vi "DisplayJson.vi"(11 "JSON String In":string="[{\"version\":\"1.0.0\",\"header\":{\"creationDate\":\"2022-06-03T00:00:00\",\"remarks\":\"\",\"serialNumber\":\"98172\",\"productNumber\":\"123021.1804\",\"productType\":\"PAA-9L\",\"pressureType\":2,\"productSeries\":\"9L\",\"compensatedTemperatureRange\":{\"min\":-10.0,\"max\":80.0,\"unit\":4},\"compensatedPressureRange\":{\"min\":0.0,\"max\":0.35,\"unit\":3},\"electricSupply\":{\"magnitude\":1.0,\"unit\":18},\"orderNumber\":9990266,\"orderPosition\":3,\"orderTargetDispatchDate\":\"2022-06-02T00:00:00+00:00\",\"customerName\":\"DemoData Inc.\",\"customerNumber\":12345678,\"customerOrderNumber\":\"Cust-9990266-123\",\"customerReferenceNumber\":\"\",\"customerProductT...") -> ()   [LabVIEW 2017] (continued)
{\"magnitude\":0.0013623391,\"unit\":7}},\"temperature\":{\"output\":{\"magnitude\":-10.8346,\"unit\":4},\"error\":{\"magnitude\":-0.10593532,\"unit\":4}}}}}},{\"reference\":\"F_12300_XX_0000098765\",\"environmentTarget\":{\"pressure\":{\"magnitude\":0.27,\"unit\":3},\"temperature\":{\"magnitude\":-10.0,\"unit\":4}},\"environment\":{\"pressure\":{\"magnitude\":0.270004,\"unit\":3},\"temperature\":{\"magnitude\":-10.7286,\"unit\":4},\"supply\":{\"magnitude\":1.0,\"unit\":18}},\"raw\":{\"signal\":{\"magnitude\":47.450500568,\"unit\":22},\"bridgeResistance\":{\"magnitude\":3280.1356798,\"unit\":28}},\"compensated\":{\"mathematicalModels\":{\"MM0123\":{\"pressure\":{\"output\":{\"magnitude\":0.27003,\"unit\":3},\"error\":{\"magnitude\":0.0074227521,\"unit\":7}},\"temperature\":{\"output\":{\"magnitude\":-10.8303,\"unit\":4},\"error\":{\"magnitude\":-0.10169503,\"unit\":4}}}}}},{\"reference\":\"F_12300_XX_0000098765\",\"environmentTarget\":{\"pressure\":{\"magnitude\":0.35,\"unit\":3},\"temperature\":{\"magnitude\":-10.0,\"unit\":4}},\"environment\":{\"pressure\":{\"magnitude\":0.350008,\"unit\":3},\"temperature\":{\"magnitude\":-10.7286,\"unit\":4},\"supply\":{\"magnitude\":1.0,\"unit\":18}},\"raw\":{\"signal\":{\"magnitude\":58.239105783,\"unit\":22},\"bridgeResistance\":{\"magnitude\":3276.3155459,\"unit\":28}},\"compensated\":{\"mathematicalModels\":{\"MM0123\":{\"pressure\":{\"output\":{\"magnitude\":0.350007,\"unit\":3},\"error\":{\"magnitude\":-0.00029844865,\"unit\":7}},\"temperature\":{\"output\":{\"magnitude\":-10.8321,\"unit\":4},\"error\":{\"magnitude\":-0.1035134,\"unit\":4}}}}}},{\"reference\":\"F_12300_XX_0000098765\",\"environmentTarget\":{\"pressure\":{\"magnitude\":0.03,\"unit\":3},\"temperature\":{\"magnitude\":0.0,\"unit\":4}},\"environment\":{\"pressure\":{\"magnitude\":0.0299972,\"unit\":3},\"temperature\":{\"magnitude\":-0.629962,\"unit\":4},\"supply\":{\"magnitude\":1.0,\"unit\":18}},\"raw\":{\"signal\":{\"magnitude\":15.244054572,\"unit\":22},\"bridgeResistance\":{\"magnitude\":3361.0174053,\"unit\":28}},\"compensated\":{\"mathematicalModels\":{\"MM0123\":{\"pressure\":{\"output\":{\"magnitude\":0.0300171,\"unit\":3},\"error\":{\"magnitude\":0.0056759296,\"unit\":7}},\"temperature\":{\"output\":{\"magnitude\":-0.733085,\"unit\":4},\"error\":{\"magnitude\":-0.10312274,\"unit\":4}}}}}},{\"reference\":\"F_12300_XX_0000098765\",\"environmentTarget\":{\"pressure\":{\"magnitude\":0.11,\"unit\":3},\"temperature\":{\"magnitude\":0.0,\"unit\":4}},\"environment\":{\"pressure\":{\"magnitude\":0.109991,\"unit\":3},\"temperature\":{\"magnitude\":-0.629962,\"unit\":4},\"supply\":{\"magnitude\":1.0,\"unit\":18}},\"raw\":{\"signal\":{\"magnitude\":26.124449139,\"unit\":22},\"bridgeResistance\":{\"magnitude\":3356.9112522,\"unit\":28}},\"compensated\":{\"mathematicalModels\":{\"MM0123\":{\"pressure\":{\"output\":{\"magnitude\":0.109967,\"unit\":3},\"error\":{\"magnitude\":-0.0069380952,\"unit\":7}},\"temperature\":{\"output\":{\"magnitude\":-0.737302,\"unit\":4},\"error\":{\"magnitude\":-0.10734013,\"unit\":4}}}}}},{\"reference\":\"F_12300_XX_0000098765\",\"environmentTarget\":{\"pressure\":{\"magnitude\":0.19,\"unit\":3},\"temperature\":{\"magnitude\":0.0,\"unit\":4}},\"environment\":{\"pressure\":{\"magnitude\":0.190002,\"unit\":3},\"temperature\":{\"magnitude\":-0.629962,\"unit\":4},\"supply\":{\"magnitude\":1.0,\"unit\":18}},\"raw\":{\"signal\":{\"magnitude\":36.977075789,\"unit\":22},\"bridgeResistance\":{\"magnitude\":3352.8969981,\"unit\":28}},\"compensated\":{\"mathematicalModels\":{\"MM0123\":{\"pressure\":{\"output\":{\"magnitude\":0.190006,\"unit\":3},\"error\":{\"magnitude\":0.0012306197,\"unit\":7}},\"temperature\":{\"output\":{\"magnitude\":-0.73875,\"unit\":4},\"error\":{\"magnitude\":-0.10878787,\"unit\":4}}}}}},{\"reference\":\"F_12300_XX_0000098765\",\"environmentTarget\":{\"pressure\":{\"magnitude\":0.27,\"unit\":3},\"temperature\":{\"magnitude\":0.0,\"unit\":4}},\"environment\":{\"pressure\":{\"magnitude\":0.269997,\"unit\":3},\"temperature\":{\"magnitude\":-0.629962,\"unit\":4},\"supply\":{\"magnitude\":1.0,\"unit\":18}},\"raw\":{\"signal\":{\"magnitude\":47.783782703,\"unit\":22},\"bridgeResistance\":{\"magnitude\":3348.9647898,\"unit\":28}},\"compensated\":{\"mathematicalModels\":{\"MM0123\":{\"pressure\":{\"output\":{\"magnitude\":0.270004,\"unit\":3},\"error\":{\"magnitude\":0.0019715764,\"unit\":7}},\"temperature\":{\"output\":{\"magnitude\":-0.74022,\"unit\":4},\"error\":{\"magnitude\":-0.11025793,\"unit\":4}}}}}},{\"reference\":\"F_12300_XX_0000098765\",\"environmentTarget\":{\"pressure\":{\"magnitude\":0.35,\"unit\":3},\"temperature\":{\"magnitude\":0.0,\"unit\":4}},\"environment\":{\"pressure\":{\"magnitude\":0.350002,\"unit\":3},\"temperature\":{\"magnitude\":-0.629962,\"unit\":4},\"supply\":{\"magnitude\":1.0,\"unit\":18}},\"raw\":{\"signal\":{\"magnitude\":58.546481606,\"unit\":22},\"bridgeResistance\":{\"magnitude\":3345.1070624,\"unit\":28}},\"compensated\":{\"mathematicalModels\":{\"MM0123\":{\"pressure\":{\"output\":{\"magnitude\":0.349974,\"unit\":3},\"error\":{\"magnitude\":-0.0079123893,\"unit\":7}},\"temperature\":{\"output\":{\"magnitude\":-0.743146,\"unit\":4},\"error\":{\"magnitude\":-0.11318368,\"unit\":4}}}}}},{\"reference\":\"F_12300_XX_0000098765\",\"environmentTarget\":{\"pressure\":{\"magnitude\":0.03,\"unit\":3},\"temperature\":{\"magnitude\":20.0,\"unit\":4}},\"environment\":{\"pressure\":{\"magnitude\":0.0300081,\"unit\":3},\"temperature\":{\"magnitude\":19.5509,\"unit\":4},\"supply\":{\"magnitude\":1.0,\"unit\":18}},\"raw\":{\"signal\":{\"magnitude\":16.125304957,\"unit\":22},\"bridgeResistance\":{\"magnitude\":3516.1742855,\"unit\":28}},\"compensated\":{\"mathematicalModels\":{\"MM0123\":{\"pressure\":{\"output\":{\"magnitude\":0.0300105,\"unit\":3},\"error\":{\"magnitude\":0.00067553345,\"unit\":7}},\"temperature\":{\"output\":{\"magnitude\":19.5453,\"unit\":4},\"error\":{\"magnitude\":-0.0056133347,\"unit\":4}}}}}},{\"reference\":\"F_12300_XX_0000098765\",\"environmentTarget\":{\"pressure\":{\"magnitude\":0.11,\"unit\":3},\"temperature\":{\"magnitude\":20.0,\"unit\":4}},\"environment\":{\"pressure\":{\"magnitude\":0.110005,\"unit\":3},\"temperature\":{\"magnitude\":19.5509,\"unit\":4},\"supply\":{\"magnitude\":1.0,\"unit\":18}},\"raw\":{\"signal\":{\"magnitude\":26.996372938,\"unit\":22},\"bridgeResistance\":{\"magnitude\":3512.074279,\"unit\":28}},\"compensated\":{\"mathematicalModels\":{\"MM0123\":{\"pressure\":{\"output\":{\"magnitude\":0.109981,\"unit\":3},\"error\":{\"magnitude\":-0.006982433,\"unit\":7}},\"temperature\":{\"output\":{\"magnitude\":19.5417,\"unit\":4},\"error\":{\"magnitude\":-0.0092010915,\"unit\":4}}}}}},{\"reference\":\"F_12300_XX_0000098765\",\"environmentTarget\":{\"pressure\":{\"magnitude\":0.19,\"unit\":3},\"temperature\":{\"magnitude\":20.0,\"unit\":4}},\"environment\":{\"pressure\":{\"magnitude\":0.19,\"unit\":3},\"temperature\":{\"magnitude\":19.5509,\"unit\":4},\"supply\":{\"magnitude\":1.0,\"unit\":18}},\"raw\":{\"signal\":{\"magnitude\":37.839811244,\"unit\":22},\"bridgeResistance\":{\"magnitude\":3508.0539307,\"unit\":28}},\"compensated\":{\"mathematicalModels\":{\"MM0123\":{\"pressure\":{\"output\":{\"magnitude\":0.190009,\"unit\":3},\"error\":{\"magnitude\":0.0025189522,\"unit\":7}},\"temperature\":{\"output\":{\"magnitude\":19.5397,\"unit\":4},\"error\":{\"magnitude\":-0.011265038,\"unit\":4}}}}}},{\"reference\":\"F_12300_XX_0000098765\",\"environmentTarget\":{\"pressure\":{\"magnitude\":0.27,\"unit\":3},\"temperature\":{\"magnitude\":20.0,\"unit\":4}},\"environment\":{\"pressure\":{\"magnitude\":0.269991,\"unit\":3},\"temperature\":{\"magnitude\":19.5509,\"unit\":4},\"supply\":{\"magnitude\":1.0,\"unit\":18}},\"raw\":{\"signal\":{\"magnitude\":48.64477597,\"unit\":22},\"bridgeResistance\":{\"magnitude\":3504.0815507,\"unit\":28}},\"compensated\":{\"mathematicalModels\":{\"MM0123\":{\"pressure\":{\"output\":{\"magnitude\":0.270017,\"unit\":3},\"error\":{\"magnitude\":0.0075196359,\"unit\":7}},\"temperature\":{\"output\":{\"magnitude\":19.5351,\"unit\":4},\"error\":{\"magnitude\":-0.015767596,\"unit\":4}}}}}},{\"reference\":\"F_12300_XX_0000098765\",\"environmentTarget\":{\"pressure\":{\"magnitude\":0.35,\"unit\":3},\"temperature\":{\"magnitude\":20.0,\"unit\":4}},\"environment\":{\"pressure\":{\"magnitude\":0.350006,\"unit\":3},\"temperature\":{\"magnitude\":19.5509,\"unit\":4},\"supply\":{\"magnitude\":1.0,\"unit\":18}},\"raw\":{\"signal\":{\"magnitude\":59.412702159,\"unit\":22},\"bridgeResistance\":{\"magnitude\":3500.1828661,\"unit\":28}},\"compensated\":{\"mathematicalModels\":{\"MM0123\":{\"pressure\":{\"output\":{\"magnitude\":0.350016,\"unit\":3},\"error\":{\"magnitude\":0.0028004951,\"unit\":7}},\"temperature\":{\"output\":{\"magnitude\":19.5311,\"unit\":4},\"error\":{\"magnitude\":-0.01974258,\"unit\":4}}}}}},{\"reference\":\"F_12300_XX_0000098765\",\"environmentTarget\":{\"pressure\":{\"magnitude\":0.03,\"unit\":3},\"temperature\":{\"magnitude\":40.0,\"unit\":4}},\"environment\":{\"pressure\":{\"magnitude\":0.0299895,\"unit\":3},\"temperature\":{\"magnitude\":39.7284,\"unit\":4},\"supply\":{\"magnitude\":1.0,\"unit\":18}},\"raw\":{\"signal\":{\"magnitude\":17.065348991,\"unit\":22},\"bridgeResistance\":{\"magnitude\":3692.0667607,\"unit\":28}},\"compensated\":{\"mathematicalModels\":{\"MM0123\":{\"pressure\":{\"output\":{\"magnitude\":0.0300063,\"unit\":3},\"error\":{\"magnitude\":0.0050974158,\"unit\":7}},\"temperature\":{\"output\":{\"magnitude\":39.7232,\"unit\":4},\"error\":{\"magnitude\":-0.0052473995,\"unit\":4}}}}}},{\"reference\":\"F_12300_XX_0000098765\",\"environmentTarget\":{\"pressure\":{\"magnitude\":0.11,\"unit\":3},\"temperature\":{\"magnitude\":40.0,\"unit\":4}},\"environment\":{\"pressure\":{\"magnitude\":0.110003,\"unit\":3},\"temperature\":{\"magnitude\":39.7284,\"unit\":4},\"supply\":{\"magnitude\":1.0,\"unit\":18}},\"raw\":{\"signal\":{\"magnitude\":27.983427862,\"unit\":22},\"bridgeResistance\":{\"magnitude\":3687.9377706,\"unit\":28}},\"compensated\":{\"mathematicalModels\":{\"MM0123\":{\"pressure\":{\"output\":{\"magnitude\":0.109977,\"unit\":3},\"error\":{\"magnitude\":-0.0073825952,\"unit\":7}},\"temperature\":{\"output\":{\"magnitude\":39.7238,\"unit\":4},\"error\":{\"magnitude\":-0.004664108,\"unit\":4}}}}}},{\"reference\":\"F_12300_XX_0000098765\",\"environmentTarget\":{\"pressure\":{\"magnitude\":0.19,\"unit\":3},\"temperature\":{\"magnitude\":40.0,\"unit\":4}},\"environment\":{\"pressure\":{\"magnitude\":0.190001,\"unit\":3},\"temperature\":{\"magnitude\":39.7284,\"unit\":4},\"supply\":{\"magnitude\":1.0,\"unit\":18}},\"raw\":{\"signal\":{\"magnitude\":38.877031412,\"unit\":22},\"bridgeResistance\":{\"magnitude\":3683.8203033,\"unit\":28}},\"compensated\":{\"mathematicalModels\":{\"MM0123\":{\"pressure\":{\"output\":{\"magnitude\":0.190002,\"unit\":3},\"error\":{\"magnitude\":0.00023079502,\"unit\":7}},\"temperature\":{\"output\":{\"magnitude\":39.7172,\"unit\":4},\"error\":{\"magnitude\":-0.011209563,\"unit\":4}}}}}},{\"reference\":\"F_12300_XX_0000098765\",\"environmentTarget\":{\"pressure\":{\"magnitude\":0.27,\"unit\":3},\"temperature\":{\"magnitude\":40.0,\"unit\":4}},\"environment\":{\"pressure\":{\"magnitude\":0.269992,\"unit\":3},\"temperature\":{\"magnitude\":39.7284,\"unit\":4},\"supply\":{\"magnitude\":1.0,\"unit\":18}},\"raw\":{\"signal\":{\"magnitude\":49.737147354,\"unit\":22},\"bridgeResistance\":{\"magnitude\":3679.8954018,\"unit\":28}},\"compensated\":{\"mathematicalModels\":{\"MM0123\":{\"pressure\":{\"output\":{\"magnitude\":0.270007,\"unit\":3},\"error\":{\"magnitude\":0.0041943925,\"unit\":7}},\"temperature\":{\"output\":{\"magnitude\":39.7218,\"unit\":4},\"error\":{\"magnitude\":-0.0066394556,\"unit\":4}}}}}},{\"reference\":\"F_12300_XX_0000098765\",\"environmentTarget\":{\"pressure\":{\"magnitude\":0.35,\"unit\":3},\"temperature\":{\"magnitude\":40.0,\"unit\":4}},\"environment\":{\"pressure\":{\"magnitude\":0.350005,\"unit\":3},\"temperature\":{\"magnitude\":39.7284,\"unit\":4},\"supply\":{\"magnitude\":1.0,\"unit\":18}},\"raw\":{\"signal\":{\"magnitude\":60.561192593,\"unit\":22},\"bridgeResistance\":{\"magnitude\":3675.9578376,\"unit\":28}},\"compensated\":{\"mathematicalModels\":{\"MM0123\":{\"pressure\":{\"output\":{\"magnitude\":0.34998,\"unit\":3},\"error\":{\"magnitude\":-0.0070559456,\"unit\":7}},\"temperature\":{\"output\":{\"magnitude\":39.7183,\"unit\":4},\"error\":{\"magnitude\":-0.010071361,\"unit\":4}}}}}},{\"reference\":\"F_12300_XX_0000098765\",\"environmentTarget\":{\"pressure\":{\"magnitude\":0.03,\"unit\":3},\"temperature\":{\"magnitude\":60.0,\"unit\":4}},\"environment\":{\"pressure\":{\"magnitude\":0.0299998,\"unit\":3},\"temperature\":{\"magnitude\":59.8651,\"unit\":4},\"supply\":{\"magnitude\":1.0,\"unit\":18}},\"raw\":{\"signal\":{\"magnitude\":18.099851195,\"unit\":22},\"bridgeResistance\":{\"magnitude\":3895.3174051,\"unit\":28}},\"compensated\":{\"mathematicalModels\":{\"MM0123\":{\"pressure\":{\"output\":{\"magnitude\":0.0300101,\"unit\":3},\"error\":{\"magnitude\":0.0029412823,\"unit\":7}},\"temperature\":{\"output\":{\"magnitude\":59.9224,\"unit\":4},\"error\":{\"magnitude\":0.057229128,\"unit\":4}}}}}},{\"reference\":\"F_12300_XX_0000098765\",\"environmentTarget\":{\"pressure\":{\"magnitude\":0.11,\"unit\":3},\"temperature\":{\"magnitude\":60.0,\"unit\":4}},\"environment\":{\"pressure\":{\"magnitude\":0.110001,\"unit\":3},\"temperature\":{\"magnitude\":59.8651,\"unit\":4},\"supply\":{\"magnitude\":1.0,\"unit\":18}},\"raw\":{\"signal\":{\"magnitude\":29.103136685,\"unit\":22},\"bridgeResistance\":{\"magnitude\":3891.1648478,\"unit\":28}},\"compensated\":{\"mathematicalModels\":{\"MM0123\":{\"pressure\":{\"output\":{\"magnitude\":0.109978,\"unit\":3},\"error\":{\"magnitude\":-0.0066748143,\"unit\":7}},\"temperature\":{\"output\":{\"magnitude\":59.9257,\"unit\":4},\"error\":{\"magnitude\":0.06060745,\"unit\":4}}}}}},{\"reference\":\"F_12300_XX_0000098765\",\"environmentTarget\":{\"pressure\":{\"magnitude\":0.19,\"unit\":3},\"temperature\":{\"magnitude\":60.0,\"unit\":4}},\"environment\":{\"pressure\":{\"magnitude\":0.190003,\"unit\":3},\"temperature\":{\"magnitude\":59.8651,\"unit\":4},\"supply\":{\"magnitude\":1.0,\"unit\":18}},\"raw\":{\"signal\":{\"magnitude\":40.086606504,\"unit\":22},\"bridgeResistance\":{\"magnitude\":3877.0460541,\"unit\":28}},\"compensated\":{\"mathematicalModels\":{\"MM0123\":{\"pressure\":{\"output\":{\"magnitude\":0.190005,\"unit\":3},\"error\":{\"magnitude\":0.00046457429,\"unit\":7}},\"temperature\":{\"output\":{\"magnitude\":59.9272,\"unit\":4},\"error\":{\"magnitude\":0.062116452,\"unit\":4}}}}}},{\"reference\":\"F_12300_XX_0000098765\",\"environmentTarget\":{\"pressure\":{\"magnitude\":0.27,\"unit\":3},\"temperature\":{\"magnitude\":60.0,\"unit\":4}},\"environment\":{\"pressure\":{\"magnitude\":0.270002,\"unit\":3},\"temperature\":{\"magnitude\":59.8651,\"unit\":4},\"supply\":{\"magnitude\":1.0,\"unit\":18}},\"raw\":{\"signal\":{\"magnitude\":51.041325527,\"unit\":22},\"bridgeResistance\":{\"magnitude\":3872.9540114,\"unit\":28}},\"compensated\":{\"mathematicalModels\":{\"MM0123\":{\"pressure\":{\"output\":{\"magnitude\":0.270027,\"unit\":3},\"error\":{\"magnitude\":0.0071406806,\"unit\":7}},\"temperature\":{\"output\":{\"magnitude\":59.9256,\"unit\":4},\"error\":{\"magnitude\":0.060455959,\"unit\":4}}}}}},{\"reference\":\"F_12300_XX_0000098765\",\"environmentTarget\":{\"pressure\":{\"magnitude\":0.35,\"unit\":3},\"temperature\":{\"magnitude\":60.0,\"unit\":4}},\"environment\":{\"pressure\":{\"magnitude\":0.349997,\"unit\":3},\"temperature\":{\"magnitude\":59.8651,\"unit\":4},\"supply\":{\"magnitude\":1.0,\"unit\":18}},\"raw\":{\"signal\":{\"magnitude\":61.960627471,\"unit\":22},\"bridgeResistance\":{\"magnitude\":3868.9899215,\"unit\":28}},\"compensated\":{\"mathematicalModels\":{\"MM0123\":{\"pressure\":{\"output\":{\"magnitude\":0.349991,\"unit\":3},\"error\":{\"magnitude\":-0.0017872561,\"unit\":7}},\"temperature\":{\"output\":{\"magnitude\":59.9305,\"unit\":4},\"error\":{\"magnitude\":0.065332416,\"unit\":4}}}}}},{\"reference\":\"F_12300_XX_0000098765\",\"environmentTarget\":{\"pressure\":{\"magnitude\":0.03,\"unit\":3},\"temperature\":{\"magnitude\":80.0,\"unit\":4}},\"environment\":{\"pressure\":{\"magnitude\":0.0300094,\"unit\":3},\"temperature\":{\"magnitude\":79.9513,\"unit\":4},\"supply\":{\"magnitude\":1.0,\"unit\":18}},\"raw\":{\"signal\":{\"magnitude\":19.261952971,\"unit\":22},\"bridgeResistance\":{\"magnitude\":4092.4016691,\"unit\":28}},\"compensated\":{\"mathematicalModels\":{\"MM0123\":{\"pressure\":{\"output\":{\"magnitude\":0.0300217,\"unit\":3},\"error\":{\"magnitude\":0.0035217854,\"unit\":7}},\"temperature\":{\"output\":{\"magnitude\":80.0395,\"unit\":4},\"error\":{\"magnitude\":0.089127618,\"unit\":4}}}}}},{\"reference\":\"F_12300_XX_0000098765\",\"environmentTarget\":{\"pressure\":{\"magnitude\":0.11,\"unit\":3},\"temperature\":{\"magnitude\":80.0,\"unit\":4}},\"environment\":{\"pressure\":{\"magnitude\":0.109996,\"unit\":3},\"temperature\":{\"magnitude\":79.9513,\"unit\":4},\"supply\":{\"magnitude\":1.0,\"unit\":18}},\"raw\":{\"signal\":{\"magnitude\":30.373856674,\"unit\":22},\"bridgeResistance\":{\"magnitude\":4089.1956244,\"unit\":28}},\"compensated\":{\"mathematicalModels\":{\"MM0123\":{\"pressure\":{\"output\":{\"magnitude\":0.109968,\"unit\":3},\"error\":{\"magnitude\":-0.0080606507,\"unit\":7}},\"temperature\":{\"output\":{\"magnitude\":80.0443,\"unit\":4},\"error\":{\"magnitude\":0.093001611,\"unit\":4}}}}}},{\"reference\":\"F_12300_XX_0000098765\",\"environmentTarget\":{\"pressure\":{\"magnitude\":0.19,\"unit\":3},\"temperature\":{\"magnitude\":80.0,\"unit\":4}},\"environment\":{\"pressure\":{\"magnitude\":0.189998,\"unit\":3},\"temperature\":{\"magnitude\":79.9513,\"unit\":4},\"supply\":{\"magnitude\":1.0,\"unit\":18}},\"raw\":{\"signal\":{\"magnitude\":41.474863124,\"unit\":22},\"bridgeResistance\":{\"magnitude\":4084.0346992,\"unit\":28}},\"compensated\":{\"mathematicalModels\":{\"MM0123\":{\"pressure\":{\"output\":{\"magnitude\":0.190001,\"unit\":3},\"error\":{\"magnitude\":0.00091335112,\"unit\":7}},\"temperature\":{\"output\":{\"magnitude\":80.0507,\"unit\":4},\"error\":{\"magnitude\":0.099395557,\"unit\":4}}}}}},{\"reference\":\"F_12300_XX_0000098765\",\"environmentTarget\":{\"pressure\":{\"magnitude\":0.27,\"unit\":3},\"temperature\":{\"magnitude\":80.0,\"unit\":4}},\"environment\":{\"pressure\":{\"magnitude\":0.270001,\"unit\":3},\"temperature\":{\"magnitude\":79.9513,\"unit\":4},\"supply\":{\"magnitude\":1.0,\"unit\":18}},\"raw\":{\"signal\":{\"magnitude\":52.55093942,\"unit\":22},\"bridgeResistance\":{\"magnitude\":4079.8926343,\"unit\":28}},\"compensated\":{\"mathematicalModels\":{\"MM0123\":{\"pressure\":{\"output\":{\"magnitude\":0.270025,\"unit\":3},\"error\":{\"magnitude\":0.0067335623,\"unit\":7}},\"temperature\":{\"output\":{\"magnitude\":80.0559,\"unit\":4},\"error\":{\"magnitude\":0.10459769,\"unit\":4}}}}}},{\"reference\":\"F_12300_XX_0000098765\",\"environmentTarget\":{\"pressure\":{\"magnitude\":0.35,\"unit\":3},\"temperature\":{\"magnitude\":80.0,\"unit\":4}},\"environment\":{\"pressure\":{\"magnitude\":0.349998,\"unit\":3},\"temperature\":{\"magnitude\":79.9513,\"unit\":4},\"supply\":{\"magnitude\":1.0,\"unit\":18}},\"raw\":{\"signal\":{\"magnitude\":63.594920576,\"unit\":22},\"bridgeResistance\":{\"magnitude\":4075.8019906,\"unit\":28}},\"compensated\":{\"mathematicalModels\":{\"MM0123\":{\"pressure\":{\"output\":{\"magnitude\":0.349986,\"unit\":3},\"error\":{\"magnitude\":-0.0033814904,\"unit\":7}},\"temperature\":{\"output\":{\"magnitude\":80.0629,\"unit\":4},\"error\":{\"magnitude\":0.11256229,\"unit\":4}}}}}}]},{\"version\":\"1.0.0\",\"header\":{\"creationDate\":\"2022-06-03T00:00:00\",\"remarks\":\"\",\"serialNumber\":\"98153\",\"productNumber\":\"123021.1804\",\"productType\":\"PAA-9L\",\"pressureType\":2,\"productSeries\":\"9L\",\"compensatedTemperatureRange\":{\"min\":-10.0,\"max\":80.0,\"unit\":4},\"compensatedPressureRange\":{\"min\":0.0,\"max\":0.35,\"unit\":3},\"electricSupply\":{\"magnitude\":1.0,\"unit\":18},\"orderNumber\":9990266,\"orderPosition\":3,\"orderTargetDispatchDate\":\"2022-06-02T00:00:00+00:00\",\"customerName\":\"DemoData Inc.\",\"customerNumber\":12345678,\"customerOrderNumber\":\"Cust-9990266-123\",\"customerReferenceNumber\":\"\",\"customerProductType\":\"123021-1804 Rev.AA\"},\"compensationMethods\":{\"mathematicalModels\":{\"MM0123\":{\"modelType\":\"MM0123\",\"productNumber\":\"000000.0000\",\"compensatedTemperatureRange\":{\"min\":-10.0,\"max\":80.0,\"unit\":4},\"compensatedPressureRange\":{\"min\":0.0,\"max\":0.35,\"unit\":3},\"electricSupply\":{\"magnitude\":1.0,\"unit\":18},\"parts\":{\"pressure\":{\"inputs\":[\"Sig\",\"R\"],\"output\":\"P\",\"description\":\"P = f(Sig,R)\",\"coefficients\":[[5.01122025899,-0.00519005490227,1.99550532962E-06,-3.43406774518E-10,2.21550439359E-14],[-0.171430315338,0.000185608282359,-7.21762353561E-08,1.24734741497E-11,-8.09638944557E-16],[0.000333004920618,-3.38999107989E-07,1.30333721973E-10,-2.23231987141E-14,1.43329122857E-18]]},\"temperature\":{\"inputs\":[\"R\",\"Sig\"],\"output\":\"T\",\"description\":\"T = f(R,Sig)\",\"coefficients\":[[-8284.8728292,22.2690862439,-0.234676407299],[8.1751505771,-0.0232330277136,0.000254914377044],[-0.00308977224278,9.12200639172E-06,-1.03722430757E-07],[5.28453653046E-07,-1.59349229999E-09,1.87313443194E-11],[-3.40890563183E-11,1.04421357223E-13,-1.26657877517E-15]]}}}}},\"measurements\":[{\"reference\":\"F_12300_XX_0000098765\",\"environmentTarget\":{\"pressure\":{\"magnitude\":0.03,\"unit\":3},\"temperature\":{\"magnitude\":-10.0,\"unit\":4}},\"environment\":{\"pressure\":{\"magnitude\":0.0299989,\"unit\":3},\"temperature\":{\"magnitude\":-10.7286,\"unit\":4},\"supply\":{\"magnitude\":1.0,\"unit\":18}},\"raw\":{\"signal\":{\"magnitude\":17.244978392,\"unit\":22},\"bridgeResistance\":{\"magnitude\":3262.0216448,\"unit\":28}},\"compensated\":{\"mathematicalModels\":{\"MM0123\":{\"pressure\":{\"output\":{\"magnitude\":0.0300081,\"unit\":3},\"error\":{\"magnitude\":0.0026236255,\"unit\":7}},\"temperature\":{\"output\":{\"magnitude\":-10.8422,\"unit\":4},\"error\":{\"magnitude\":-0.11354536,\"unit\":4}}}}}},{\"reference\":\"F_12300_XX_0000098765\",\"environmentTarget\":{\"pressure\":{\"magnitude\":0.11,\"unit\":3},\"temperature\":{\"magnitude\":-10.0,\"unit\":4}},\"environment\":{\"pressure\":{\"magnitude\":0.109995,\"unit\":3},\"temperature\":{\"magnitude\":-10.7286,\"unit\":4},\"supply\":{\"magnitude\":1.0,\"unit\":18}},\"raw\":{\"signal\":{\"magnitude\":28.068610601,\"unit\":22},\"bridgeResistance\":{\"magnitude\":3257.9781268,\"unit\":28}},\"compensated\":{\"mathematicalModels\":{\"MM0123\":{\"pressure\":{\"output\":{\"magnitude\":0.109969,\"unit\":3},\"error\":{\"magnitude\":-0.0075611348,\"unit\":7}},\"temperature\":{\"output\":{\"magnitude\":-10.8372,\"unit\":4},\"error\":{\"magnitude\":-0.10860353,\"unit\":4}}}}}},{\"reference\":\"F_12300_XX_0000098765\",\"environmentTarget\":{\"pressure\":{\"magnitude\":0.19,\"unit\":3},\"temperature\":{\"magnitude\":-10.0,\"unit\":4}},\"environment\":{\"pressure\":{\"magnitude\":0.190006,\"unit\":3},\"temperature\":{\"magnitude\":-10.7286,\"unit\":4},\"supply\":{\"magnitude\":1.0,\"unit\":18}},\"raw\":{\"signal\":{\"magnitude\":38.861396244,\"unit\":22},\"bridgeResistance\":{\"magnitude\":3253.9392,\"unit\":28}},\"compensated\":{\"mathematicalModels\":{\"MM0123\":{\"pressure\":{\"output\":{\"magnitude\":0.190014,\"unit\":3},\"error\":{\"magnitude\":0.0022942891,\"unit\":7}},\"temperature\":{\"output\":{\"magnitude\":-10.8453,\"unit\":4},\"error\":{\"magnitude\":-0.11664439,\"unit\":4}}}}}},{\"reference\":\"F_12300_XX_0000098765\",\"environmentTarget\":{\"pressure\":{\"magnitude\":0.27,\"unit\":3},\"temperature\":{\"magnitude\":-10.0,\"unit\":4}},\"environment\":{\"pressure\":{\"magnitude\":0.270007,\"unit\":3},\"temperature\":{\"magnitude\":-10.7286,\"unit\":4},\"supply\":{\"magnitude\":1.0,\"unit\":18}},\"raw\":{\"signal\":{\"magnitude\":49.608942701,\"unit\":22},\"bridgeResistance\":{\"magnitude\":3250.0878585,\"unit\":28}},\"compensated\":{\"mathematicalModels\":{\"MM0123\":{\"pressure\":{\"output\":{\"magnitude\":0.270032,\"unit\":3},\"error\":{\"magnitude\":0.0071075807,\"unit\":7}},\"temperature\":{\"output\":{\"magnitude\":-10.84,\"unit\":4},\"error\":{\"magnitude\":-0.11234415,\"unit\":4}}}}}},{\"reference\":\"F_12300_XX_0000098765\",\"environmentTarget\":{\"pressure\":{\"magnitude\":0.35,\"unit\":3},\"temperature\":{\"magnitude\":-10.0,\"unit\":4}},\"environment\":{\"pressure\":{\"magnitude\":0.350003,\"unit\":3},\"temperature\":{\"magnitude\":-10.7286,\"unit\":4},\"supply\":{\"magnitude\":1.0,\"unit\":18}},\"raw\":{\"signal\":{\"magnitude\":60.306965463,\"unit\":22},\"bridgeResistance\":{\"magnitude\":3246.287526,\"unit\":28}},\"compensated\":{\"mathematicalModels\":{\"MM0123\":{\"pressure\":{\"output\":{\"magnitude\":0.35,\"unit\":3},\"error\":{\"magnitude\":-0.00094624232,\"unit\":7}},\"temperature\":{\"output\":{\"magnitude\":-10.8431,\"unit\":4},\"error\":{\"magnitude\":-0.11441768,\"unit\":4}}}}}},{\"reference\":\"F_12300_XX_0000098765\",\"environmentTarget\":{\"pressure\":{\"magnitude\":0.03,\"unit\":3},\"temperature\":{\"magnitude\":0.0,\"unit\":4}},\"environment\":{\"pressure\":{\"magnitude\":0.0299957,\"unit\":3},\"temperature\":{\"magnitude\":-0.629962,\"unit\":4},\"supply\":{\"magnitude\":1.0,\"unit\":18}},\"raw\":{\"signal\":{\"magnitude\":17.697410923,\"unit\":22},\"bridgeResistance\":{\"magnitude\":3330.8433823,\"unit\":28}},\"compensated\":{\"mathematicalModels\":{\"MM0123\":{\"pressure\":{\"output\":{\"magnitude\":0.0300103,\"unit\":3},\"error\":{\"magnitude\":0.0041629875,\"unit\":7}},\"temperature\":{\"output\":{\"magnitude\":-0.740686,\"unit\":4},\"error\":{\"magnitude\":-0.11072407,\"unit\":4}}}}}},{\"reference\":\"F_12300_XX_0000098765\",\"environmentTarget\":{\"pressure\":{\"magnitude\":0.11,\"unit\":3},\"temperature\":{\"magnitude\":0.0,\"unit\":4}},\"environment\":{\"pressure\":{\"magnitude\":0.109989,\"unit\":3},\"temperature\":{\"magnitude\":-0.629962,\"unit\":4},\"supply\":{\"magnitude\":1.0,\"unit\":18}},\"raw\":{\"signal\":{\"magnitude\":28.4892745,\"unit\":22},\"bridgeResistance\":{\"magnitude\":3326.7612608,\"unit\":28}},\"compensated\":{\"mathematicalModels\":{\"MM0123\":{\"pressure\":{\"output\":{\"magnitude\":0.109964,\"unit\":3},\"error\":{\"magnitude\":-0.0070954752,\"unit\":7}},\"temperature\":{\"output\":{\"magnitude\":-0.747272,\"unit\":4},\"error\":{\"magnitude\":-0.11731048,\"unit\":4}}}}}},{\"reference\":\"F_12300_XX_0000098765\",\"environmentTarget\":{\"pressure\":{\"magnitude\":0.19,\"unit\":3},\"temperature\":{\"magnitude\":0.0,\"unit\":4}},\"environment\":{\"pressure\":{\"magnitude\":0.190002,\"unit\":3},\"temperature\":{\"magnitude\":-0.629962,\"unit\":4},\"supply\":{\"magnitude\":1.0,\"unit\":18}},\"raw\":{\"signal\":{\"magnitude\":39.252857819,\"unit\":22},\"bridgeResistance\":{\"magnitude\":3322.8054195,\"unit\":28}},\"compensated\":{\"mathematicalModels\":{\"MM0123\":{\"pressure\":{\"output\":{\"magnitude\":0.189998,\"unit\":3},\"error\":{\"magnitude\":-0.0011297609,\"unit\":7}},\"temperature\":{\"output\":{\"magnitude\":-0.746289,\"unit\":4},\"error\":{\"magnitude\":-0.11632608,\"unit\":4}}}}}},{\"reference\":\"F_12300_XX_0000098765\",\"environmentTarget\":{\"pressure\":{\"magnitude\":0.27,\"unit\":3},\"temperature\":{\"magnitude\":0.0,\"unit\":4}},\"environment\":{\"pressure\":{\"magnitude\":0.269998,\"unit\":3},\"temperature\":{\"magnitude\":-0.629962,\"unit\":4},\"supply\":{\"magnitude\":1.0,\"unit\":18}},\"raw\":{\"signal\":{\"magnitude\":49.973804513,\"unit\":22},\"bridgeResistance\":{\"magnitude\":3318.899856,\"unit\":28}},\"compensated\":{\"mathematicalModels\":{\"MM0123\":{\"pressure\":{\"output\":{\"magnitude\":0.27001,\"unit\":3},\"error\":{\"magnitude\":0.0034989265,\"unit\":7}},\"temperature\":{\"output\":{\"magnitude\":-0.749528,\"unit\":4},\"error\":{\"magnitude\":-0.11956623,\"unit\":4}}}}}},{\"reference\":\"F_12300_XX_0000098765\",\"environmentTarget\":{\"pressure\":{\"magnitude\":0.35,\"unit\":3},\"temperature\":{\"magnitude\":0.0,\"unit\":4}},\"environment\":{\"pressure\":{\"magnitude\":0.350006,\"unit\":3},\"temperature\":{\"magnitude\":-0.629962,\"unit\":4},\"supply\":{\"magnitude\":1.0,\"unit\":18}},\"raw\":{\"signal\":{\"magnitude\":60.649198409,\"unit\":22},\"bridgeResistance\":{\"magnitude\":3315.0808233,\"unit\":28}},\"compensated\":{\"mathematicalModels\":{\"MM0123\":{\"pressure\":{\"output\":{\"magnitude\":0.349978,\"unit\":3},\"error\":{\"magnitude\":-0.0079789618,\"unit\":7}},\"temperature\":{\"output\":{\"magnitude\":-0.752383,\"unit\":4},\"error\":{\"magnitude\":-0.12242084,\"unit\":4}}}}}},{\"reference\":\"F_12300_XX_0000098765\",\"environmentTarget\":{\"pressure\":{\"magnitude\":0.03,\"unit\":3},\"temperature\":{\"magnitude\":20.0,\"unit\":4}},\"environment\":{\"pressure\":{\"magnitude\":0.029999,\"unit\":3},\"temperature\":{\"magnitude\":19.5509,\"unit\":4},\"supply\":{\"magnitude\":1.0,\"unit\":18}},\"raw\":{\"signal\":{\"magnitude\":18.650570403,\"unit\":22},\"bridgeResistance\":{\"magnitude\":3485.7702276,\"unit\":28}},\"compensated\":{\"mathematicalModels\":{\"MM0123\":{\"pressure\":{\"output\":{\"magnitude\":0.0300063,\"unit\":3},\"error\":{\"magnitude\":0.0020803458,\"unit\":7}},\"temperature\":{\"output\":{\"magnitude\":19.5415,\"unit\":4},\"error\":{\"magnitude\":-0.0093833592,\"unit\":4}}}}}},{\"reference\":\"F_12300_XX_0000098765\",\"environmentTarget\":{\"pressure\":{\"magnitude\":0.11,\"unit\":3},\"temperature\":{\"magnitude\":20.0,\"unit\":4}},\"environment\":{\"pressure\":{\"magnitude\":0.110002,\"unit\":3},\"temperature\":{\"magnitude\":19.5509,\"unit\":4},\"supply\":{\"magnitude\":1.0,\"unit\":18}},\"raw\":{\"signal\":{\"magnitude\":29.437602066,\"unit\":22},\"bridgeResistance\":{\"magnitude\":3481.7140234,\"unit\":28}},\"compensated\":{\"mathematicalModels\":{\"MM0123\":{\"pressure\":{\"output\":{\"magnitude\":0.109982,\"unit\":3},\"error\":{\"magnitude\":-0.0057937112,\"unit\":7}},\"temperature\":{\"output\":{\"magnitude\":19.5392,\"unit\":4},\"error\":{\"magnitude\":-0.011651533,\"unit\":4}}}}}},{\"reference\":\"F_12300_XX_0000098765\",\"environmentTarget\":{\"pressure\":{\"magnitude\":0.19,\"unit\":3},\"temperature\":{\"magnitude\":20.0,\"unit\":4}},\"environment\":{\"pressure\":{\"magnitude\":0.190002,\"unit\":3},\"temperature\":{\"magnitude\":19.5509,\"unit\":4},\"supply\":{\"magnitude\":1.0,\"unit\":18}},\"raw\":{\"signal\":{\"magnitude\":40.196372991,\"unit\":22},\"bridgeResistance\":{\"magnitude\":3477.715328,\"unit\":28}},\"compensated\":{\"mathematicalModels\":{\"MM0123\":{\"pressure\":{\"output\":{\"magnitude\":0.19001,\"unit\":3},\"error\":{\"magnitude\":0.0023661198,\"unit\":7}},\"temperature\":{\"output\":{\"magnitude\":19.5357,\"unit\":4},\"error\":{\"magnitude\":-0.015193505,\"unit\":4}}}}}},{\"reference\":\"F_12300_XX_0000098765\",\"environmentTarget\":{\"pressure\":{\"magnitude\":0.27,\"unit\":3},\"temperature\":{\"magnitude\":20.0,\"unit\":4}},\"environment\":{\"pressure\":{\"magnitude\":0.269995,\"unit\":3},\"temperature\":{\"magnitude\":19.5509,\"unit\":4},\"supply\":{\"magnitude\":1.0,\"unit\":18}},\"raw\":{\"signal\":{\"magnitude\":50.917814334,\"unit\":22},\"bridgeResistance\":{\"magnitude\":3473.7940622,\"unit\":28}},\"compensated\":{\"mathematicalModels\":{\"MM0123\":{\"pressure\":{\"output\":{\"magnitude\":0.270024,\"unit\":3},\"error\":{\"magnitude\":0.0082649059,\"unit\":7}},\"temperature\":{\"output\":{\"magnitude\":19.5329,\"unit\":4},\"error\":{\"magnitude\":-0.017941357,\"unit\":4}}}}}},{\"reference\":\"F_12300_XX_0000098765\",\"environmentTarget\":{\"pressure\":{\"magnitude\":0.35,\"unit\":3},\"temperature\":{\"magnitude\":20.0,\"unit\":4}},\"environment\":{\"pressure\":{\"magnitude\":0.350007,\"unit\":3},\"temperature\":{\"magnitude\":19.5509,\"unit\":4},\"supply\":{\"magnitude\":1.0,\"unit\":18}},\"raw\":{\"signal\":{\"magnitude\":61.600753754,\"unit\":22},\"bridgeResistance\":{\"magnitude\":3469.9282528,\"unit\":28}},\"compensated\":{\"mathematicalModels\":{\"MM0123\":{\"pressure\":{\"output\":{\"magnitude\":0.350015,\"unit\":3},\"error\":{\"magnitude\":0.002212532,\"unit\":7}},\"temperature\":{\"output\":{\"magnitude\":19.5283,\"unit\":4},\"error\":{\"magnitude\":-0.022578737,\"unit\":4}}}}}},{\"reference\":\"F_12300_XX_0000098765\",\"environmentTarget\":{\"pressure\":{\"magnitude\":0.03,\"unit\":3},\"temperature\":{\"magnitude\":40.0,\"unit\":4}},\"environment\":{\"pressure\":{\"magnitude\":0.0300029,\"unit\":3},\"temperature\":{\"magnitude\":39.7284,\"unit\":4},\"supply\":{\"magnitude\":1.0,\"unit\":18}},\"raw\":{\"signal\":{\"magnitude\":19.689183227,\"unit\":22},\"bridgeResistance\":{\"magnitude\":3660.9751606,\"unit\":28}},\"compensated\":{\"mathematicalModels\":{\"MM0123\":{\"pressure\":{\"output\":{\"magnitude\":0.0300171,\"unit\":3},\"error\":{\"magnitude\":0.004062793,\"unit\":7}},\"temperature\":{\"output\":{\"magnitude\":39.7238,\"unit\":4},\"error\":{\"magnitude\":-0.0046353676,\"unit\":4}}}}}},{\"reference\":\"F_12300_XX_0000098765\",\"environmentTarget\":{\"pressure\":{\"magnitude\":0.11,\"unit\":3},\"temperature\":{\"magnitude\":40.0,\"unit\":4}},\"environment\":{\"pressure\":{\"magnitude\":0.110002,\"unit\":3},\"temperature\":{\"magnitude\":39.7284,\"unit\":4},\"supply\":{\"magnitude\":1.0,\"unit\":18}},\"raw\":{\"signal\":{\"magnitude\":30.524706124,\"unit\":22},\"bridgeResistance\":{\"magnitude\":3656.8762185,\"unit\":28}},\"compensated\":{\"mathematicalModels\":{\"MM0123\":{\"pressure\":{\"output\":{\"magnitude\":0.109977,\"unit\":3},\"error\":{\"magnitude\":-0.0071312014,\"unit\":7}},\"temperature\":{\"output\":{\"magnitude\":39.7238,\"unit\":4},\"error\":{\"magnitude\":-0.0045700104,\"unit\":4}}}}}},{\"reference\":\"F_12300_XX_0000098765\",\"environmentTarget\":{\"pressure\":{\"magnitude\":0.19,\"unit\":3},\"temperature\":{\"magnitude\":40.0,\"unit\":4}},\"environment\":{\"pressure\":{\"magnitude\":0.190005,\"unit\":3},\"temperature\":{\"magnitude\":39.7284,\"unit\":4},\"supply\":{\"magnitude\":1.0,\"unit\":18}},\"raw\":{\"signal\":{\"magnitude\":41.337078939,\"unit\":22},\"bridgeResistance\":{\"magnitude\":3652.7974978,\"unit\":28}},\"compensated\":{\"mathematicalModels\":{\"MM0123\":{\"pressure\":{\"output\":{\"magnitude\":0.190002,\"unit\":3},\"error\":{\"magnitude\":-0.00072364867,\"unit\":7}},\"temperature\":{\"output\":{\"magnitude\":39.718,\"unit\":4},\"error\":{\"magnitude\":-0.0103739,\"unit\":4}}}}}},{\"reference\":\"F_12300_XX_0000098765\",\"environmentTarget\":{\"pressure\":{\"magnitude\":0.27,\"unit\":3},\"temperature\":{\"magnitude\":40.0,\"unit\":4}},\"environment\":{\"pressure\":{\"magnitude\":0.269992,\"unit\":3},\"temperature\":{\"magnitude\":39.7284,\"unit\":4},\"supply\":{\"magnitude\":1.0,\"unit\":18}},\"raw\":{\"signal\":{\"magnitude\":52.115466737,\"unit\":22},\"bridgeResistance\":{\"magnitude\":3648.891645,\"unit\":28}},\"compensated\":{\"mathematicalModels\":{\"MM0123\":{\"pressure\":{\"output\":{\"magnitude\":0.270006,\"unit\":3},\"error\":{\"magnitude\":0.004101221,\"unit\":7}},\"temperature\":{\"output\":{\"magnitude\":39.7215,\"unit\":4},\"error\":{\"magnitude\":-0.0068958529,\"unit\":4}}}}}},{\"reference\":\"F_12300_XX_0000098765\",\"environmentTarget\":{\"pressure\":{\"magnitude\":0.35,\"unit\":3},\"temperature\":{\"magnitude\":40.0,\"unit\":4}},\"environment\":{\"pressure\":{\"magnitude\":0.350002,\"unit\":3},\"temperature\":{\"magnitude\":39.7284,\"unit\":4},\"supply\":{\"magnitude\":1.0,\"unit\":18}},\"raw\":{\"signal\":{\"magnitude\":62.857601327,\"unit\":22},\"bridgeResistance\":{\"magnitude\":3644.9865367,\"unit\":28}},\"compensated\":{\"mathematicalModels\":{\"MM0123\":{\"pressure\":{\"output\":{\"magnitude\":0.349979,\"unit\":3},\"error\":{\"magnitude\":-0.0067115071,\"unit\":7}},\"temperature\":{\"output\":{\"magnitude\":39.7187,\"unit\":4},\"error\":{\"magnitude\":-0.0097278689,\"unit\":4}}}}}},{\"reference\":\"F_12300_XX_0000098765\",\"environmentTarget\":{\"pressure\":{\"magnitude\":0.03,\"unit\":3},\"temperature\":{\"magnitude\":60.0,\"unit\":4}},\"environment\":{\"pressure\":{\"magnitude\":0.0300019,\"unit\":3},\"temperature\":{\"magnitude\":59.8651,\"unit\":4},\"supply\":{\"magnitude\":1.0,\"unit\":18}},\"raw\":{\"signal\":{\"magnitude\":20.839840408,\"unit\":22},\"bridgeResistance\":{\"magnitude\":3853.2059511,\"unit\":28}},\"compensated\":{\"mathematicalModels\":{\"MM0123\":{\"pressure\":{\"output\":{\"magnitude\":0.0300114,\"unit\":3},\"error\":{\"magnitude\":0.0027075586,\"unit\":7}},\"temperature\":{\"output\":{\"magnitude\":59.9284,\"unit\":4},\"error\":{\"magnitude\":0.063301799,\"unit\":4}}}}}},{\"reference\":\"F_12300_XX_0000098765\",\"environmentTarget\":{\"pressure\":{\"magnitude\":0.11,\"unit\":3},\"temperature\":{\"magnitude\":60.0,\"unit\":4}},\"environment\":{\"pressure\":{\"magnitude\":0.110001,\"unit\":3},\"temperature\":{\"magnitude\":59.8651,\"unit\":4},\"supply\":{\"magnitude\":1.0,\"unit\":18}},\"raw\":{\"signal\":{\"magnitude\":31.763522286,\"unit\":22},\"bridgeResistance\":{\"magnitude\":3849.07117,\"unit\":28}},\"compensated\":{\"mathematicalModels\":{\"MM0123\":{\"pressure\":{\"output\":{\"magnitude\":0.10998,\"unit\":3},\"error\":{\"magnitude\":-0.0059063219,\"unit\":7}},\"temperature\":{\"output\":{\"magnitude\":59.9307,\"unit\":4},\"error\":{\"magnitude\":0.065589004,\"unit\":4}}}}}},{\"reference\":\"F_12300_XX_0000098765\",\"environmentTarget\":{\"pressure\":{\"magnitude\":0.19,\"unit\":3},\"temperature\":{\"magnitude\":60.0,\"unit\":4}},\"environment\":{\"pressure\":{\"magnitude\":0.190013,\"unit\":3},\"temperature\":{\"magnitude\":59.8651,\"unit\":4},\"supply\":{\"magnitude\":1.0,\"unit\":18}},\"raw\":{\"signal\":{\"magnitude\":42.66874911,\"unit\":22},\"bridgeResistance\":{\"magnitude\":3844.9896596,\"unit\":28}},\"compensated\":{\"mathematicalModels\":{\"MM0123\":{\"pressure\":{\"output\":{\"magnitude\":0.190016,\"unit\":3},\"error\":{\"magnitude\":0.00090499253,\"unit\":7}},\"temperature\":{\"output\":{\"magnitude\":59.9327,\"unit\":4},\"error\":{\"magnitude\":0.067575032,\"unit\":4}}}}}},{\"reference\":\"F_12300_XX_0000098765\",\"environmentTarget\":{\"pressure\":{\"magnitude\":0.27,\"unit\":3},\"temperature\":{\"magnitude\":60.0,\"unit\":4}},\"environment\":{\"pressure\":{\"magnitude\":0.270007,\"unit\":3},\"temperature\":{\"magnitude\":59.8651,\"unit\":4},\"supply\":{\"magnitude\":1.0,\"unit\":18}},\"raw\":{\"signal\":{\"magnitude\":53.543034,\"unit\":22},\"bridgeResistance\":{\"magnitude\":3840.951531,\"unit\":28}},\"compensated\":{\"mathematicalModels\":{\"MM0123\":{\"pressure\":{\"output\":{\"magnitude\":0.270029,\"unit\":3},\"error\":{\"magnitude\":0.006189455,\"unit\":7}},\"temperature\":{\"output\":{\"magnitude\":59.9328,\"unit\":4},\"error\":{\"magnitude\":0.067622428,\"unit\":4}}}}}},{\"reference\":\"F_12300_XX_0000098765\",\"environmentTarget\":{\"pressure\":{\"magnitude\":0.35,\"unit\":3},\"temperature\":{\"magnitude\":60.0,\"unit\":4}},\"environment\":{\"pressure\":{\"magnitude\":0.349993,\"unit\":3},\"temperature\":{\"magnitude\":59.8651,\"unit\":4},\"supply\":{\"magnitude\":1.0,\"unit\":18}},\"raw\":{\"signal\":{\"magnitude\":64.382718571,\"unit\":22},\"bridgeResistance\":{\"magnitude\":3837.009158,\"unit\":28}},\"compensated\":{\"mathematicalModels\":{\"MM0123\":{\"pressure\":{\"output\":{\"magnitude\":0.349989,\"unit\":3},\"error\":{\"magnitude\":-0.001417396,\"unit\":7}},\"temperature\":{\"output\":{\"magnitude\":59.9359,\"unit\":4},\"error\":{\"magnitude\":0.070746414,\"unit\":4}}}}}},{\"reference\":\"F_12300_XX_0000098765\",\"environmentTarget\":{\"pressure\":{\"magnitude\":0.03,\"unit\":3},\"temperature\":{\"magnitude\":80.0,\"unit\":4}},\"environment\":{\"pressure\":{\"magnitude\":0.0300034,\"unit\":3},\"temperature\":{\"m
